vi "Create.vi"(8 "error in (no error)":errorcluster) -> (0 "error out":errorcluster, 3 "Test Result Handler":refnum<class "TestStand Result Handler.lvclass">)   [LabVIEW 2020, in "Astemes_CSVReportPlugin.lvlib" / "TestStand Result Handler.lvclass"]
uses:
  TestStand Result Handler.lvclass
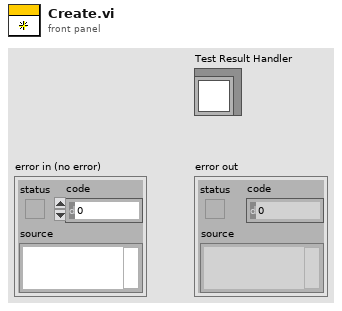
[diagram p1: front panel]
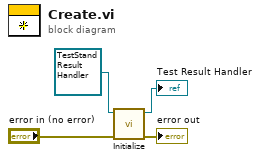
[diagram p0: block diagram]
diagram:
  n1 = call "Initialize.vi"("error in (no error)"="error in (no error)", "TestStand Result Handler in"=refnum<class "TestStand Result Handler.lvclass"> refnum ("Test Result Handler 2")) -> ("error out"=→"error out":errorcluster, "TestStand Result Handler out"=→"Test Result Handler":refnum<class "TestStand Result Handler.lvclass">)  [unwired: 8 in]
